vi "Load XML.vi"(8 "error in":errorcluster, 10 "path to XML document":path, 11 "XML Document in":refnum<class "XML Document.lvclass">) -> (0 "error out":errorcluster, 3 "XML Document out":refnum<class "XML Document.lvclass">)   [LabVIEW 2014, in "XML Document.lvclass"]
uses:
  XML Document.lvclass
  <vilib>/xml/Load XML File.vi
  <vilib>/xml/NI_XML.lvlib
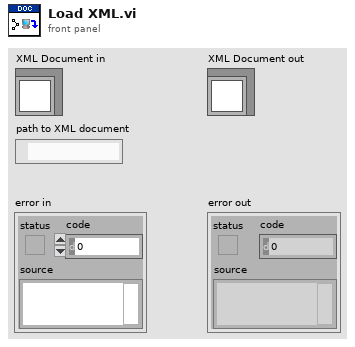
[diagram p1: front panel]
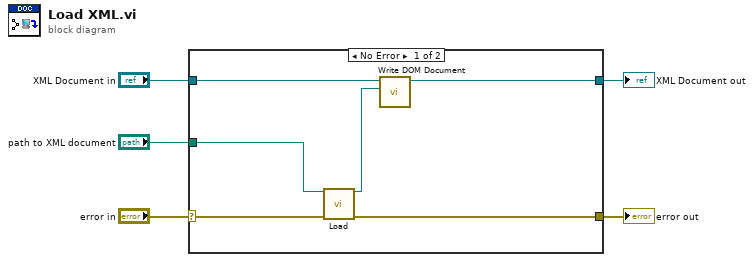
[diagram p0: block diagram]
diagram:
  n1 = case shown="No Error" "error in" {
    selector: "error in" -> [w7 w13]
    tunnel: [w6 w13] -> w4
    tunnel: [w9 w12] -> w2
    tunnel: "XML Document in" -> [w11 w12]
    tunnel: "path to XML document" -> [w10 _]
    frame No Error {
      n2 = call-poly <vilib>:"Load.vi"("path to XML document"=w10, "error in (no error)"=w7) -> ("DOM document out"=w8:refnum<k20>, "error out"=w6:errorcluster)  [unwired: 11 in, 1 out]
      n3 = call-dynamic "Write DOM Document.vi"("DOM Document"=w8, "XML Document in"=w11) -> ("XML Document out"=w9:refnum<class "XML Document.lvclass">)  [unwired: 8 in, 1 out]
    }
    frame Error {
    }
  }
  "error out" <- w4
  "XML Document out" <- w2
